vi "Serial Error Handler.vi"(8 "error in (no error)":errorcluster) -> (0 "error out":errorcluster)   [LabVIEW 2018, in "ASI TG-1000.lvlib"]
uses:
  ASI TG-1000.lvlib
  <vilib>/Utility/error.llb/DialogType.ctl
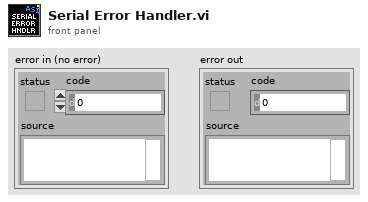
[diagram p1: front panel]
types:
  T1 = typedef "DialogType.ctl" = u16
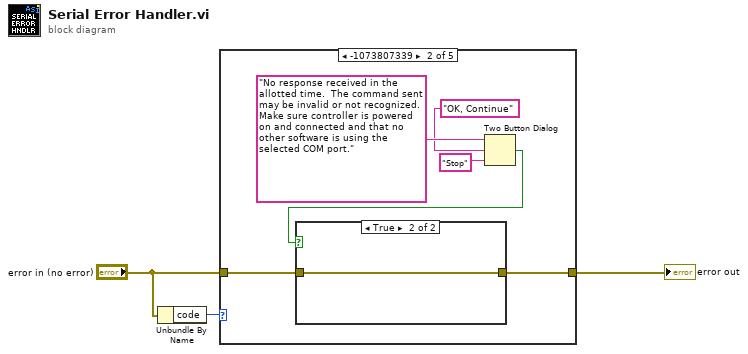
[diagram p0: block diagram]
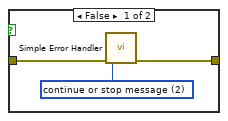
[diagram p3: hidden frame]
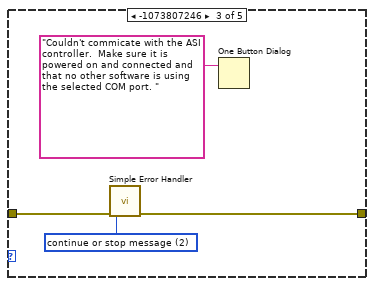
[diagram p4: hidden frame]
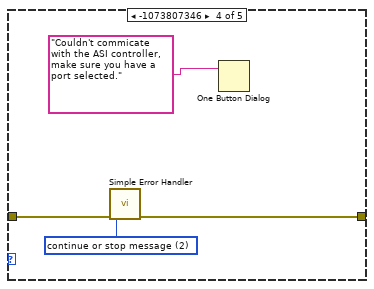
[diagram p5: hidden frame]
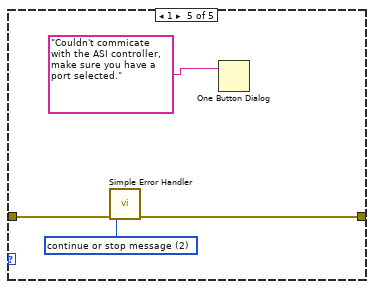
[diagram p6: hidden frame]
diagram:
  n1 = Unbundle By Name("error in (no error)") -> ("code"=w1:i32)
  n2 = case shown="-1073807339" w1 {
    tunnel: "error in (no error)" -> [w4 w9 w17 w22 w26]
    tunnel: [w4 w8 w16 w21 w25] -> w3
    frame Default {
    }
    frame -1073807339 {
      n3 = Two Button Dialog(message="No response received in the allotted time.  The command sent may be invalid or not recognized.  Make sure controller is powered on and connected and that no other software is using the selected COM port.", 1:"Stop" ("F button name (\"Cancel\")"), 2:"OK, Continue" ("T button name (\"OK\")")) -> (T button?=w5:bool)
      n4 = case shown="True" w5 {
        tunnel: w9 -> [w13 w14]
        tunnel: [w12 w14] -> w8
        frame False {
          w11 = T1 2 items=["no dialog", "OK message", "continue or stop message", "OK message + warnings", "continue/stop + warnings"] ("type of dialog (OK msg:1)")
          n5 = call <vilib>:"Simple Error Handler.vi"("type of dialog (OK msg:1)"=w11, "error in (no error)"=w13) -> ("error out"=w12:errorcluster)  [unwired: 3 in, 4 out]
        }
        frame True {
        }
      }
    }
    frame -1073807246 {
      w15 = T1 2 items=["no dialog", "OK message", "continue or stop message", "OK message + warnings", "continue/stop + warnings"] ("type of dialog (OK msg:1)")
      n6 = call <vilib>:"Simple Error Handler.vi"("type of dialog (OK msg:1)"=w15, "error in (no error)"=w17) -> ("error out"=w16:errorcluster)  [unwired: 3 in, 4 out]
      n7 = One Button Dialog(message="Couldn't commicate with the ASI controller.  Make sure it is powered on and connected and that no other software is using the selected COM port. ") -> ()  [unwired: 1 in, 1 out]
    }
    frame -1073807346 {
      w20 = T1 2 items=["no dialog", "OK message", "continue or stop message", "OK message + warnings", "continue/stop + warnings"] ("type of dialog (OK msg:1)")
      n8 = call <vilib>:"Simple Error Handler.vi"("type of dialog (OK msg:1)"=w20, "error in (no error)"=w22) -> ("error out"=w21:errorcluster)  [unwired: 3 in, 4 out]
      n9 = One Button Dialog(message="Couldn't commicate with the ASI controller, make sure you have a port selected.") -> ()  [unwired: 1 in, 1 out]
    }
    frame 1 {
      w24 = T1 2 items=["no dialog", "OK message", "continue or stop message", "OK message + warnings", "continue/stop + warnings"] ("type of dialog (OK msg:1)")
      n10 = call <vilib>:"Simple Error Handler.vi"("type of dialog (OK msg:1)"=w24, "error in (no error)"=w26) -> ("error out"=w25:errorcluster)  [unwired: 3 in, 4 out]
      n11 = One Button Dialog(message="Couldn't commicate with the ASI controller, make sure you have a port selected.") -> ()  [unwired: 1 in, 1 out]
    }
  }
  "error out" <- w3
